vi "Configure Limit Line.vi"(0 "VISA resource name":refnum<visa-resource-name>, 1 "Vertical Axis Limit Line (1:Relative)":i32(ring)=1 items=["Fixed/ABS", "Relative"], 2 "Horizontal Axis Limit Line (1:Relative)":i32(ring)=1 items=["Fixed/ABS", "Relative"], 3 "Previous Pt Level Offset":dbl[](array[numeric]), 5 "Limit Line (1)":i32=1 min=1 max=6, 7 "Limit Line Type (0:Upper)":i32(ring) items=["Upper", "Lower"], 9 "Enable Limit Line Display (F:Disable)":bool, 11 "error in (no error)":errorcluster, 12 "Enable Offset Margin State (F:Disable)":bool, 13 "Margin (0.00dB)":dbl, 14 "Enable Mirror Limit (F:Disable)":bool) -> (4 "VISA resource name out":refnum<visa-resource-name>, 15 "error out":errorcluster)   [LabVIEW 2020, in "Anritsu Signal Analyzer Series.lvlib"]
doc: "Configures the envelope settings of the spectrum analyzer."
uses:
  Anritsu Signal Analyzer Series.lvlib
panel:
  # "dB"
  # "dB"
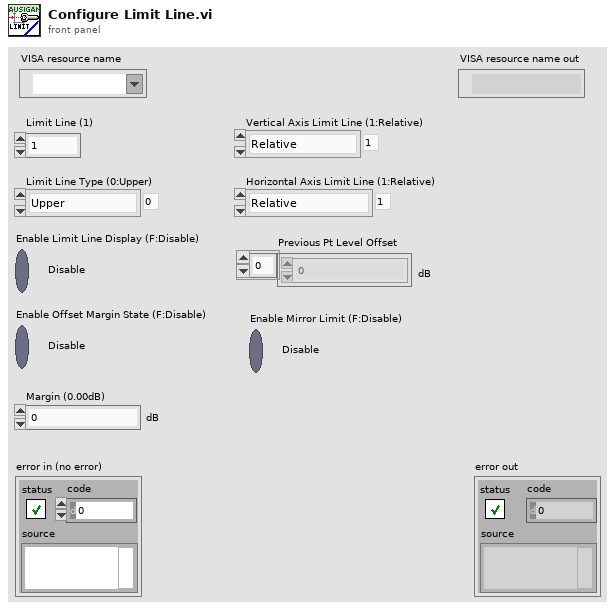
[diagram p1: front panel]
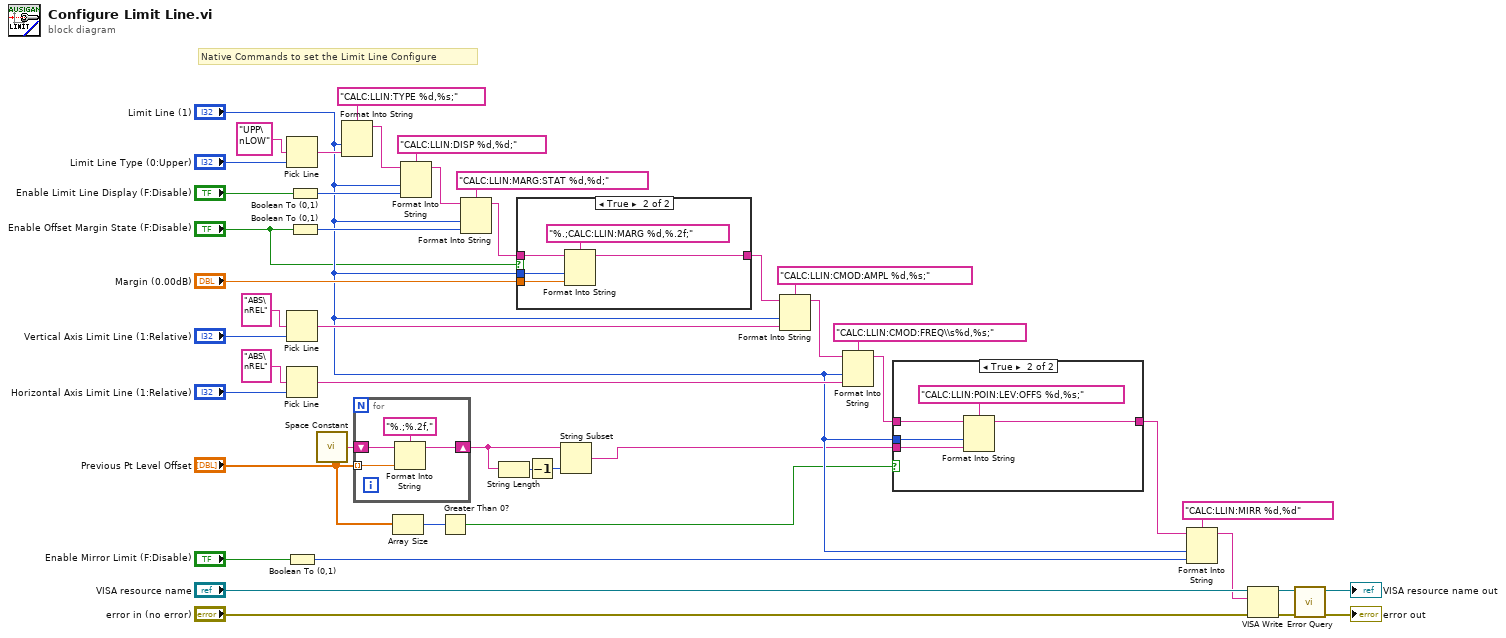
[diagram p0: block diagram]
diagram:
  # "Native Commands to set the Limit Line Configure"
  n1 = Pick Line(multi-line string="UPP\nLOW" ("複数行文字列"), line index="Limit Line Type (0:Upper)") -> (output string=w38:string)  [unwired: 1 in]
  n2 = Pick Line(multi-line string="ABS\nREL" ("複数行文字列"), line index="Vertical Axis Limit Line (1:Relative)") -> (output string=w22:string)  [unwired: 1 in]
  n3 = Pick Line(multi-line string="ABS\nREL" ("複数行文字列"), line index="Horizontal Axis Limit Line (1:Relative)") -> (output string=w20:string)  [unwired: 1 in]
  n4 = Boolean To (0,1)(Boolean="Enable Mirror Limit (F:Disable)") -> (0, 1=w13:i16)
  n5 = Boolean To (0,1)(Boolean="Enable Limit Line Display (F:Disable)") -> (0, 1=w33:i16)
  n6 = Boolean To (0,1)(Boolean="Enable Offset Margin State (F:Disable)") -> (0, 1=w30:i16)
  n7 = call <vilib>:"Space Constant.vi"() -> ("String"=w17:string)
  n8 = Format Into String(format string="CALC:LLIN:TYPE %d,%s;", "Limit Line (1)", w38) -> (resulting string=w9:string)  [unwired: 2 in, 1 out]
  n9 = for {
    tunnel: "Previous Pt Level Offset" -> [w48] mode=indexing
    shift-right: [w46] -> w3
    shift-left: w17 -> [w47]
    n10 = Format Into String(format string="%.;%.2f,", initial string=w47, w48) -> (resulting string=w46:string)  [unwired: 1 in, 1 out]
  }
  n11 = Array Size(array="Previous Pt Level Offset") -> (size(s)=w7:i32)
  n12 = Format Into String(format string="CALC:LLIN:DISP %d,%d;", initial string=w9, "Limit Line (1)", w33) -> (resulting string=w27:string)  [unwired: 1 in, 1 out]
  n13 = Greater Than 0?(x=w7) -> (x > 0?=w6:bool)
  n14 = Format Into String(format string="CALC:LLIN:MARG:STAT %d,%d;", initial string=w27, "Limit Line (1)", w30) -> (resulting string=w26:string)  [unwired: 1 in, 1 out]
  n15 = String Length(string=w3) -> (length=w5:i32)
  n16 = case shown="True" "Enable Offset Margin State (F:Disable)" {
    tunnel: "Margin (0.00dB)" -> [_ w54]
    tunnel: w26 -> [w50 w53]
    tunnel: [w50 w52] -> w23
    tunnel: "Limit Line (1)" -> [_ w51]
    frame False {
    }
    frame True {
      n17 = Format Into String(format string="%.;CALC:LLIN:MARG %d,%.2f;", initial string=w53, w51, w54) -> (resulting string=w52:string)  [unwired: 1 in, 1 out]
    }
  }
  n18 = Decrement(x=w5) -> (x-1=w4:i32)
  n19 = String Subset(string=w3, length (rest)=w4) -> (substring=w2:string)  [unwired: 1 in]
  n20 = Format Into String(format string="CALC:LLIN:CMOD:AMPL %d,%s;", initial string=w23, "Limit Line (1)", w22) -> (resulting string=w11:string)  [unwired: 1 in, 1 out]
  n21 = Format Into String(format string="CALC:LLIN:CMOD:FREQ\\s%d,%s;", initial string=w11, "Limit Line (1)", w20) -> (resulting string=w18:string)  [unwired: 1 in, 1 out]
  n22 = case shown="True" w6 {
    tunnel: w18 -> [w56 w61]
    tunnel: w2 -> [_ w59]
    tunnel: "Limit Line (1)" -> [_ w58]
    tunnel: [w56 w57] -> w15
    frame False {
    }
    frame True {
      n23 = Format Into String(format string="CALC:LLIN:POIN:LEV:OFFS %d,%s;", initial string=w61, w58, w59) -> (resulting string=w57:string)  [unwired: 1 in, 1 out]
    }
  }
  n24 = Format Into String(format string="CALC:LLIN:MIRR %d,%d", initial string=w15, "Limit Line (1)", w13) -> (resulting string=w1:string)  [unwired: 1 in, 1 out]
  n25 = VISA Write(VISA resource name="VISA resource name", write buffer=w1, error in (no error)="error in (no error)") -> (VISA resource name out=w41:refnum<visa-resource-name>, error out=w40:errorcluster)  [unwired: 1 out]
  n26 = call "Error Query.vi"("error in (no error)"=w40, "VISA resource name"=w41) -> ("error out"=→"error out":errorcluster, "VISA resource name out"=→"VISA resource name out":refnum<visa-resource-name>)  [unwired: 6 in, 2 out]
